vi "Global 224.vi"() -> ()   [LabVIEW 2013]
panel:
  out "Beam ON":bool
  in  "NMR Channel":i32=2 min=0 max=7 step=1
  in  "TEQ Comment":string="Unused"
  in  "Q Comment":string="Unused"
  in  "TEQ file":string="NMRave.xls"
  in  "Measurement":enum16{"TEQ", "POL", "QCV"}(ring)
  in  "Commentary":string="213 MHz crystal, SMT03 RF Gen"
  in  "Calib Constant":dbl=1.0 min=0.0 max=1.0 step=0.001 format="%_3f"
  out "File name":string="C:\\users\\plm\\Desktop\\rssmt\\data\\TEQ3559333835.csv"
  in  "IP Address":string="192.168.0.4"
  in  "Gain":enum16{"LOW", "HI", "MAX"}(ring)=enum."MAX"
  in  "COM Port #":refnum<visa-resource-name>="COM8"
  out "Peak center (MHz)":sgl=224.47049 format="%.3f"
  in  "Logoffset (V)":dbl=-5.38 min=-9.0 max=0.0 step=0.0005 format="%_5g"
  in  "Phase (V)":dbl=7.3 min=0.0 max=10.7 step=0.0005 format="%_5g"
  in  "Real/Quad Q curve":bool=TRUE
  out "Temperature (C)":dbl(graph)=25.88
  out "+3V supply":dbl=3.294 format="%_4g"
  out "Temp (C)":dbl=25.88 format="%_4g"
  in  "RemovePed":bool=TRUE
  in  "IF / LOG Det":bool
  in  "Q curve file":string="NMRave.xls"
  in  "AutoTune":bool=TRUE
  out "RF OK":bool=TRUE
  out "Peak area (mV-MHz)":sgl=4.069452 format="%.5f"
  in  "Gauss Fit":bool
  out "NMR Graph + Fit":cluster{cluster{dbl, "Numeric":dbl}[]}[](graph)=[{[{224.37, "Numeric"=-0.004794050000003608}, {224.371, "Numeric"=-0.005454050000001955}, {224.372, "Numeric"=-0.005117450000000332}, {224.373, "Numeric"=-0.0037842500000081682}, {224.374, "Numeric"=-0.005454450000006519}, {224.375, "Numeric"=-0.0051280500000048974}, {224.376, "Numeric"=-0.005805050000003312}, {224.377, "Numeric"=-0.005485450000001758}, {224.37800000000001, "Numeric"=-0.005169250000000236}, {224.379, "Numeric"=-0.00585645000000759}, {224.38, "Numeric"=-0.005547050000006035}, {224.381, "Numeric"=-0.005241050000004514}, {224.382, "Numeric"=-0.004938450000003026}, {224.383, "Numeric"=-0.004639250000001569}, {224.38400000000001, "Numeric"=-0.005343450000000145}, {224.385, "Numeric"=-0.005051050000007017}, {224.386, "Numeric"=-0.004762050000005562}, {224.387, "Numeric"=-0.004476450000004139}, {224.388, "Numeric"=-0.004194250000002748}, {224.389, "Numeric"=-0.003915450000001389}, {224.39000000000001, "Numeric"=-0.0036400500000000648}, {224.391, "Numeric"=-0.004368050000006453}, {224.392, "Numeric"=-0.0030994500000050967}, {224.393, "Numeric"=-0.003834250000003772}, {224.394, "Numeric"=-0.0035724500000024802}, {224.395, "Numeric"=-0.00331405000000122}, {224.39600000000002, "Numeric"=-0.004059049999999995}, {224.397, "Numeric"=-0.002807450000005901}, {224.398, "Numeric"=-0.002559250000004641}, {224.399, "Numeric"=-0.003314450000003414}, {224.4, "Numeric"=-0.0030730500000022212}, {224.401, "Numeric"=-0.0038350500000010595}, {224.40200000000002, "Numeric"=-0.00460044999999993}, {224.403, "Numeric"=-0.003369250000005354}, {224.404, "Numeric"=-0.003141450000004195}, {224.405, "Numeric"=-0.003917050000003067}, {224.406, "Numeric"=-0.00369605000000197}, {224.407, "Numeric"=-0.0034784500000009065}, {224.40800000000002, "Numeric"=-0.0032642499999998766}, {224.409, "Numeric"=-0.0030534500000048218}, {224.41, "Numeric"=-0.0028460500000037584}, {224.411, "Numeric"=-0.002642050000002727}, {224.412, "Numeric"=-0.0024414500000017308}, {224.413, "Numeric"=-0.003244250000000764}, {224.41400000000002, "Numeric"=-0.0020504499999998323}, {224.415, "Numeric"=-0.0018600500000042954}, {224.416, "Numeric"=-0.0016730500000033312}, {224.417, "Numeric"=-0.0004894500000023998}, {224.418, "Numeric"=-0.0003092500000014993}, {224.419, "Numeric"=-0.0001324500000006324}, {224.42000000000002, "Numeric"=4.095000000020263e-05}, {224.421, "Numeric"=0.00021094999999621972}, {224.422, "Numeric"=0.00037754999999708647}, {224.423, "Numeric"=0.0005407499999979214}, {224.424, "Numeric"=0.0007005499999987227}, {224.425, "Numeric"=0.0018569499999994913}, {224.426, "Numeric"=0.002009950000000227}, {224.427, "Numeric"=0.002159549999996728}, {224.428, "Numeric"=0.0023057499999974956}, {224.429, "Numeric"=0.0024485499999982313}, {224.43, "Numeric"=0.004587949999998934}, {224.431, "Numeric"=0.0047239499999996055}, {224.432, "Numeric"=0.003856550000000243}, {224.433, "Numeric"=0.003985749999997226}, {224.434, "Numeric"=0.004111549999997895}, {224.435, "Numeric"=0.004233949999998533}, {224.436, "Numeric"=0.005352949999999138}, {224.437, "Numeric"=0.00646854999999971}, {224.438, "Numeric"=0.00658075000000025}, {224.439, "Numeric"=0.0066895499999977135}, {224.44, "Numeric"=0.007794949999998285}, {224.441, "Numeric"=0.008896949999998825}, {224.442, "Numeric"=0.010995549999999332}, {224.443, "Numeric"=0.012090749999999807}, {224.444, "Numeric"=0.013182550000000248}, {224.445, "Numeric"=0.015270949999998193}, {224.446, "Numeric"=0.017355949999998666}, {224.447, "Numeric"=0.01943754999999911}, {224.448, "Numeric"=0.021515749999999514}, {224.449, "Numeric"=0.02359054999999989}, {224.45, "Numeric"=0.02566195000000024}, {224.451, "Numeric"=0.02772994999999866}, {224.452, "Numeric"=0.02979454999999904}, {224.453, "Numeric"=0.03385574999999938}, {224.454, "Numeric"=0.03791354999999969}, {224.455, "Numeric"=0.04196794999999997}, {224.456, "Numeric"=0.04701895000000021}, {224.457, "Numeric"=0.05306654999999912}, {224.458, "Numeric"=0.0591107499999994}, {224.459, "Numeric"=0.06615154999999964}, {224.46, "Numeric"=0.07518894999999987}, {224.461, "Numeric"=0.08422295000000005}, {224.462, "Numeric"=0.09425355000000019}, {224.463, "Numeric"=0.10328074999999956}, {224.464, "Numeric"=0.11430454999999975}, {224.465, "Numeric"=0.1253249499999999}, {224.466, "Numeric"=0.13834195000000002}, {224.467, "Numeric"=0.1483555500000001}, {224.468, "Numeric"=0.15636575000000014}, {224.469, "Numeric"=0.16237255000000003}, {224.47, "Numeric"=0.1643759500000001}, {224.471, "Numeric"=0.16237595000000016}, {224.472, "Numeric"=0.15837255000000017}, {224.47299999999998, "Numeric"=0.14936575000000016}, {224.474, "Numeric"=0.1403555500000001}, {224.475, "Numeric"=0.13134195000000046}, {224.476, "Numeric"=0.12132495000000043}, {224.477, "Numeric"=0.10930455000000039}, {224.478, "Numeric"=0.0982807500000003}, {224.47899999999998, "Numeric"=0.09025355000000018}, {224.48, "Numeric"=0.08122295000000004}, {224.481, "Numeric"=0.07418895000000086}, {224.482, "Numeric"=0.06615155000000075}, {224.483, "Numeric"=0.06011075000000061}, {224.484, "Numeric"=0.05506655000000043}, {224.48499999999999, "Numeric"=0.051018950000000216}, {224.486, "Numeric"=0.045967949999999966}, {224.487, "Numeric"=0.041913550000001285}, {224.488, "Numeric"=0.03885575000000108}, {224.489, "Numeric"=0.03579455000000083}, {224.49, "Numeric"=0.03272995000000055}, {224.49099999999999, "Numeric"=0.029661950000000235}, {224.492, "Numeric"=0.02759054999999989}, {224.493, "Numeric"=0.02551575000000169}, {224.494, "Numeric"=0.025437550000001377}, {224.495, "Numeric"=0.024355950000001035}, {224.496, "Numeric"=0.022270950000000657}, {224.49699999999999, "Numeric"=0.021182550000000248}, {224.498, "Numeric"=0.019090750000002463}, {224.499, "Numeric"=0.017995550000002084}, {224.5, "Numeric"=0.015896950000001676}, {224.501, "Numeric"=0.014794950000001233}, {224.502, "Numeric"=0.014689550000000759}, {224.503, "Numeric"=0.01358075000000025}, {224.504, "Numeric"=0.012468550000002947}, {224.505, "Numeric"=0.011352950000002473}, {224.506, "Numeric"=0.010233950000001962}, {224.507, "Numeric"=0.010111550000001423}, {224.508, "Numeric"=0.00998575000000085}, {224.509, "Numeric"=0.009856550000000243}, {224.51, "Numeric"=0.009723950000003423}, {224.511, "Numeric"=0.008587950000002849}, {224.512, "Numeric"=0.008448550000002242}, {224.513, "Numeric"=0.008305750000001604}, {224.514, "Numeric"=0.007159550000000932}, {224.515, "Numeric"=0.006009950000000227}, {224.516, "Numeric"=0.005856950000003888}, {224.517, "Numeric"=0.005700550000003217}, {224.518, "Numeric"=0.005540750000002511}, {224.519, "Numeric"=0.005377550000001774}, {224.51999999999998, "Numeric"=0.005210950000001004}, {224.521, "Numeric"=0.005040950000000202}, {224.522, "Numeric"=0.004867550000004344}, {224.523, "Numeric"=0.004690750000003573}, {224.524, "Numeric"=0.004510550000002771}, {224.525, "Numeric"=0.0043269500000019355}, {224.52599999999998, "Numeric"=0.0041399500000010685}, {224.527, "Numeric"=0.003949550000000168}, {224.528, "Numeric"=0.002755750000004791}, {224.529, "Numeric"=0.003558550000003923}, {224.53, "Numeric"=0.003357950000003022}, {224.531, "Numeric"=0.0031539500000020877}, {224.53199999999998, "Numeric"=0.0029465500000011215}, {224.533, "Numeric"=0.0027357500000001235}, {224.534, "Numeric"=0.0035215500000052294}, {224.535, "Numeric"=0.003303950000004262}, {224.536, "Numeric"=0.003082950000003263}, {224.537, "Numeric"=0.0028585500000022305}, {224.53799999999998, "Numeric"=0.002630750000001167}, {224.539, "Numeric"=0.0023995500000000697}, {224.54, "Numeric"=0.0021649500000056575}, {224.541, "Numeric"=0.002926950000004592}, {224.542, "Numeric"=0.0026855500000034947}, {224.543, "Numeric"=0.0014407500000023655}, {224.54399999999998, "Numeric"=0.002192550000001202}, {224.545, "Numeric"=0.0019409500000000073}, {224.546, "Numeric"=0.001685950000006077}, {224.547, "Numeric"=0.0014275500000049124}, {224.548, "Numeric"=0.001165750000003716}, {224.549, "Numeric"=0.0009005500000024876}, {224.54999999999998, "Numeric"=0.00163195000000123}, {224.551, "Numeric"=0.0013599499999999362}, {224.552, "Numeric"=0.0010845500000064862}, {224.553, "Numeric"=-0.000194249999994775}, {224.554, "Numeric"=0.0015235500000039294}, {224.555, "Numeric"=0.0022379500000026045}, {224.55599999999998, "Numeric"=0.000948950000001246}, {224.557, "Numeric"=0.0006565499999998566}, {224.558, "Numeric"=0.0003607500000068868}, {224.559, "Numeric"=0.0010615500000055265}, {224.56, "Numeric"=0.0007589500000041351}, {224.561, "Numeric"=0.00045295000000271195}, {224.56199999999998, "Numeric"=0.0011435500000012526}, {224.563, "Numeric"=0.0008307499999997657}, {224.564, "Numeric"=0.0005145500000072779}, {224.565, "Numeric"=0.0011949500000058202}, {224.566, "Numeric"=0.0018719500000043306}, {224.567, "Numeric"=0.0015455500000028065}, {224.56799999999998, "Numeric"=0.0012157500000012506}, {224.569, "Numeric"=0.0008825499999996662}, {224.57, "Numeric"=0.0015459500000076613}]}]
  in  "Amp of Q curve":dbl=1.7000000000000004 min=0.0 max=1000.0 step=0.01 format="%_3f"
  in  "Subtract Q curve":bool=TRUE
  out "Pedestal Offset":dbl(graph)=-0.010376375000000125
  out "Pedestal Difference":dbl(graph)=0.005839700000005656
  out "# Good Spectra":i32=988
  in  "Quality cuts":bool=TRUE
  out "Pedestal OK":bool=TRUE
  out "Sweep #":i32=13
  out "1st Sweep":bool
  out "ADC volts OK":bool=TRUE
  out "Peak Height Distribution":cluster{"Y":dbl[], "Y":dbl[]}[](graph)=[{"Y"=[0.042160036666668343, 0.04219720333333501, 0.04223437000000167, 0.042271536666668344, 0.04230870333333501, 0.04234587000000167, 0.042383036666668344, 0.04242020333333501, 0.042457370000001673, 0.042494536666668345, 0.04253170333333501, 0.042568870000001674, 0.04260603666666834, 0.04264320333333501, 0.042680370000001674, 0.04271753666666834, 0.04275470333333501, 0.042791870000001675, 0.04282903666666834, 0.04286620333333501, 0.042903370000001675, 0.04294053666666834, 0.04297770333333501, 0.043014870000001676, 0.04305203666666834, 0.04308920333333501, 0.043126370000001676, 0.04316353666666834, 0.04320070333333501, 0.04323787000000168, 0.04327503666666834, 0.04331220333333501, 0.04334937000000168, 0.04338653666666834, 0.04342370333333501, 0.04346087000000168, 0.04349803666666834, 0.04353520333333501, 0.04357237000000168, 0.04360953666666834, 0.04364670333333501, 0.04368387000000168, 0.04372103666666834, 0.04375820333333501, 0.04379537000000168, 0.043832536666668344, 0.04386970333333501, 0.04390687000000168, 0.043944036666668344, 0.04398120333333501, 0.04401837000000168, 0.044055536666668345, 0.04409270333333501, 0.04412987000000168, 0.044167036666668345, 0.04420420333333501, 0.04424137000000168, 0.044278536666668346, 0.04431570333333501, 0.04435287000000168, 0.044390036666668346, 0.04442720333333501, 0.044464370000001675, 0.04450153666666835, 0.04453870333333501, 0.044575870000001676, 0.04461303666666835, 0.04465020333333501, 0.044687370000001676, 0.04472453666666835, 0.04476170333333501, 0.04479887000000168, 0.04483603666666835, 0.04487320333333501, 0.04491037000000168, 0.04494753666666835, 0.04498470333333501, 0.04502187000000168, 0.04505903666666835, 0.045096203333335014, 0.04513337000000168, 0.04517053666666835, 0.045207703333335014, 0.04524487000000168, 0.04528203666666835, 0.045319203333335015, 0.04535637000000168, 0.045393536666668344, 0.045430703333335015, 0.04546787000000168, 0.045505036666668344, 0.045542203333335016, 0.04557937000000168, 0.045616536666668345, 0.045653703333335016, 0.04569087000000168, 0.045728036666668345, 0.04576520333333502, 0.04580237000000168, 0.045839536666668346], "Y"=[1.0, 1.0, 2.0, 3.0, 2.0, 3.0, 3.0, 0.0, 5.0, 1.0, 3.0, 3.0, 2.0, 5.0, 2.0, 6.0, 5.0, 8.0, 4.0, 11.0, 8.0, 3.0, 10.0, 8.0, 12.0, 9.0, 13.0, 16.0, 18.0, 6.0, 12.0, 7.0, 12.0, 14.0, 22.0, 18.0, 12.0, 10.0, 17.0, 18.0, 19.0, 24.0, 19.0, 19.0, 18.0, 20.0, 20.0, 29.0, 14.0, 12.0, 14.0, 18.0, 23.0, 19.0, 19.0, 11.0, 19.0, 17.0, 16.0, 26.0, 25.0, 8.0, 12.0, 15.0, 8.0, 22.0, 19.0, 16.0, 8.0, 13.0, 16.0, 12.0, 11.0, 6.0, 7.0, 9.0, 12.0, 5.0, 10.0, 5.0, 7.0, 4.0, 5.0, 3.0, 5.0, 5.0, 4.0, 4.0, 1.0, 2.0, 2.0, 3.0, 1.0, 2.0, 3.0, 1.0, 2.0, 1.0, 2.0, 1.0]}]
  in  "# of Sweeps":i32=1000
  out "S/N":dbl=60.56893184534198 format="%_3g"
  out "Peak mean (V)":dbl=0.04397488788124324 format="%_4g"
  out "Peak Height":dbl(graph)=0.1643759500000001
  in  "Raw Data":bool=TRUE
  in  "Tank RF":bool=TRUE
  out "IF Atten (dB)":i8=10 min=0 max=31 step=1
  in  "IFoffset (V)":dbl=4.00575000000007 min=-0.0 max=9.0 step=0.001 format="%.4f"
  in  "Tune  (V)":dbl=2.3319999999999967 min=-0.5 max=8.0 step=0.001 format="%.4f"
  in  "Invert Polarity":bool=TRUE
  out "Pedestal Diff (V)":sgl=0.0058397 format="%.3f"
  out "Peak amp (V)":sgl=0.16437595 format="%.4f"
  in  "Save Data to File":bool=TRUE
  out "RF Level (dBm)":dbl=9.0 min=-10.0 max=10.0 step=0.1 format="%.2f"
  out "Sample RMS (V)":dbl format="%.4f"
  in  "# Sample/step":i32=20 min=1 max=1000 step=1
  in  "Step Width (MHz)":dbl=0.001 min=0.0 max=1000.0 step=5e-05 format="%.5f"
  in  "Freq Span (MHz)":dbl=0.2 min=0.0 max=50.0 step=0.1 format="%.3f"
  in  "Center Freq (MHz)":dbl=224.47 min=150.0 max=250.0 step=0.1 format="%.3f"
  # "Settings"
  # "E1039 Global NMR Control Panel"
  # "R\nF\n\nG\nE\nN \n\n+\n\nI\nF"
  # "D\nA\nC\ns"
  # "A\nD\nC"
  # "I\n/\nO"
  # "D\nA\nT\nA\n\nA \nN\nA\nL\nY\nS\nI\nS"
  # "Polarization"
  # "/ Polarization %"
  # "Results"
  # "A\nv\ne\nr\na\ng\ne\ns"
  # "S\nw\ne\ne\np"
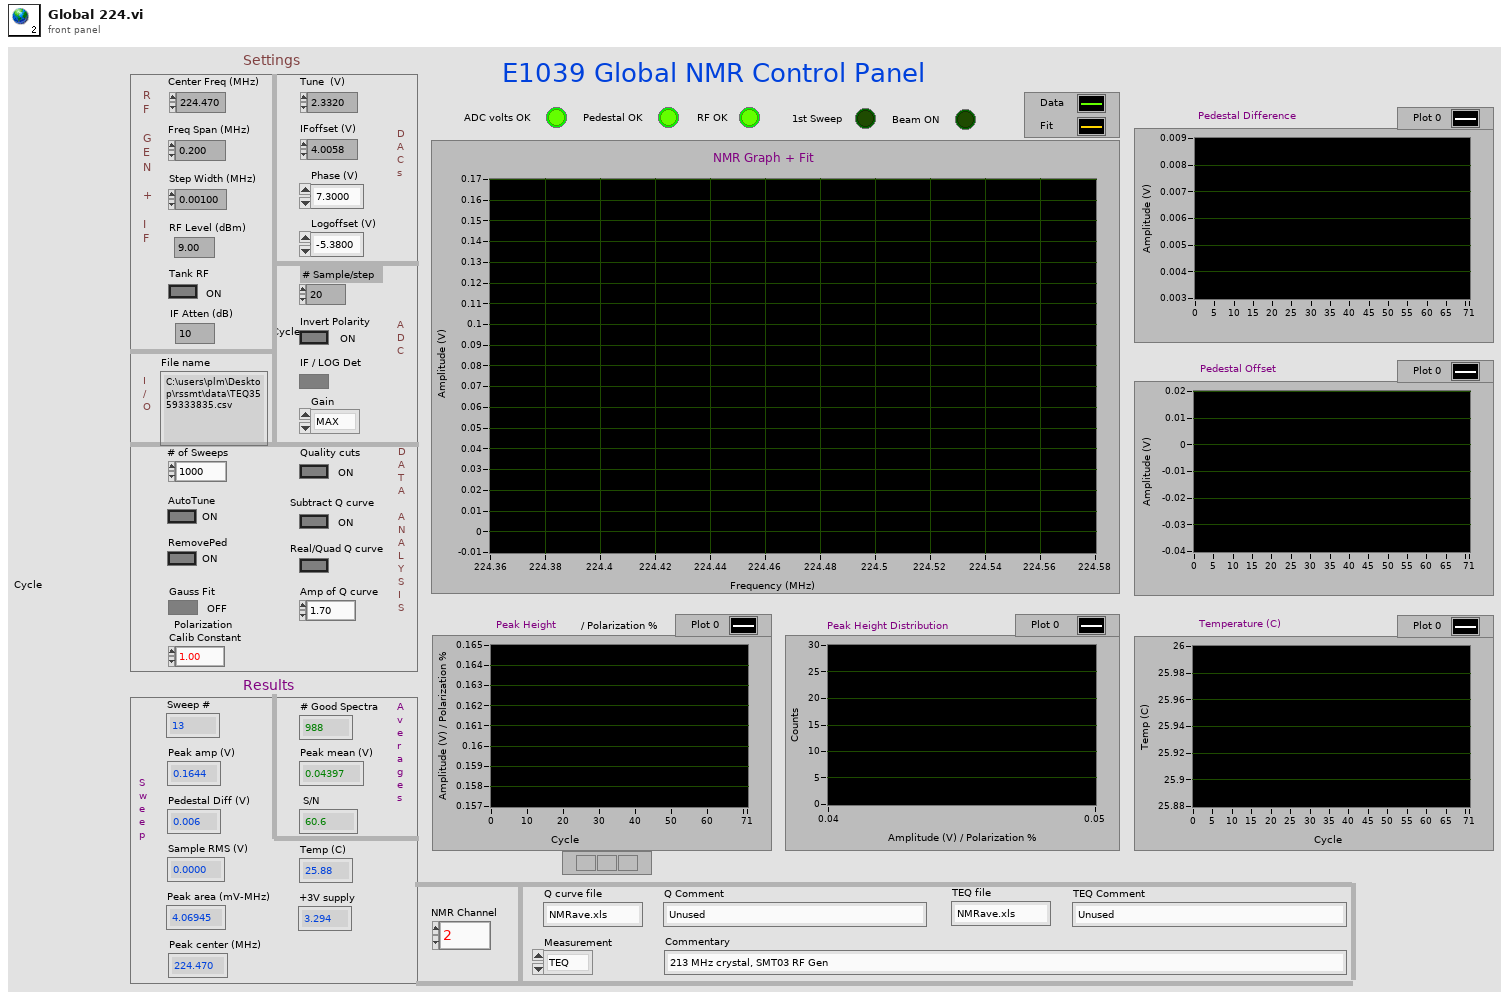
[diagram p1: front panel]
diagram:
